vi "Transfer Group.Set Direction.vi"(10 "Direction":T1, 11 "Transfer Group in":refnum<class "Transfer Group.lvclass">) -> (3 "Transfer Group out":refnum<class "Transfer Group.lvclass">)   [LabVIEW 2017, in "DSF.Engine.lvlib" / "Transfer Group.lvclass"]
uses:
  Transfer Group.lvclass
  DSF Configuration API/1.0.0/Public/Controls/DSF Direction.ctl
  Transfer Group.lvclass/Transfer Group.ctl
  DSF Configuration API/1.0.0/DSF Configuration API.lvlib
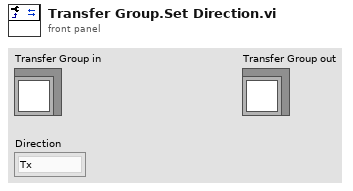
[diagram p1: front panel]
types:
  T1 = typedef "DSF Configuration API.lvlib/DSF Direction.ctl" = enum8{"Tx", "Rx"}
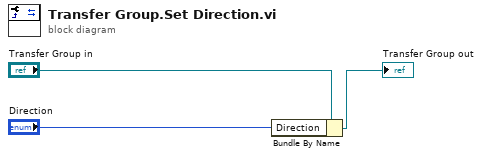
[diagram p0: block diagram]
diagram:
  n1 = Bundle By Name(cluster="Transfer Group in", "Direction"="Direction") -> (→"Transfer Group out":refnum<class "Transfer Group.lvclass">)
